vi "Sort Scan Parameters.vi"(8 "error in (no error)":errorcluster, 11 "SweepControl":refnum<class "SweepControl.lvclass">) -> (0 "error out":errorcluster, 1 "Sorted scan parameters":cluster{T1}[](array[cluster])=[{[{"Start"=0.14, "End"=-0.060000000000000005, "Step"=-0.060000000000000005, "Rate"=0.0, "wait (ms)"=10000, "Address"="Dev2/ao0", "channel"=1}]}, {[{"Start"=0.14, "End"=-0.060000000000000005, "Step"=-0.060000000000000005, "Rate"=0.0, "wait (ms)"=10000, "Address"="Dev2/ao0", "channel"=1}]}, {[{"Start"=0.14, "End"=-0.060000000000000005, "Step"=-0.060000000000000005, "Rate"=0.0, "wait (ms)"=10000, "Address"="Dev2/ao0", "channel"=1}, {"Start"=0.14, "End"=-0.060000000000000005, "Step"=-0.060000000000000005, "Rate"=0.0, "wait (ms)"=10000, "Address"="Dev2/ao0", "channel"=1}]}] {"?"."Rate" format="%.2f"; "?"."Step" format="%#_6p"; "?"."End" format="%#_6p"; "?"."Start" format="%#_6p"}, 2 "Sorted scan control":cluster{T3}[](array[cluster])=[{[{"Priority"=enum."Priority 0", "Scan name"=enum."DSA_Vsg2"}]}, {[{"Priority"=enum."Priority 1", "Scan name"=enum."DSA_Vamp"}]}, {[{"Priority"=enum."Priority 2", "Scan name"=enum."DSA_Vsg1"}, {"Priority"=enum."Priority 2", "Scan name"=enum."DSA_Vsg3"}]}], 3 "SweepControl":refnum<class "SweepControl.lvclass">)   [LabVIEW 2016, in "SweepControl.lvclass"]
uses:
  SweepControl.lvclass
  Typedefs/ScanControl.ctl
  Typedefs/Cluster - ScanControl.ctl
  Typedefs/Enum - Priority.ctl
  Typedefs/Enum - Action.ctl
  Typedefs/ScanParamters.ctl
  Typedefs/Cluster - ScanParamters.ctl
  SweepControl.lvclass/SweepControl.ctl
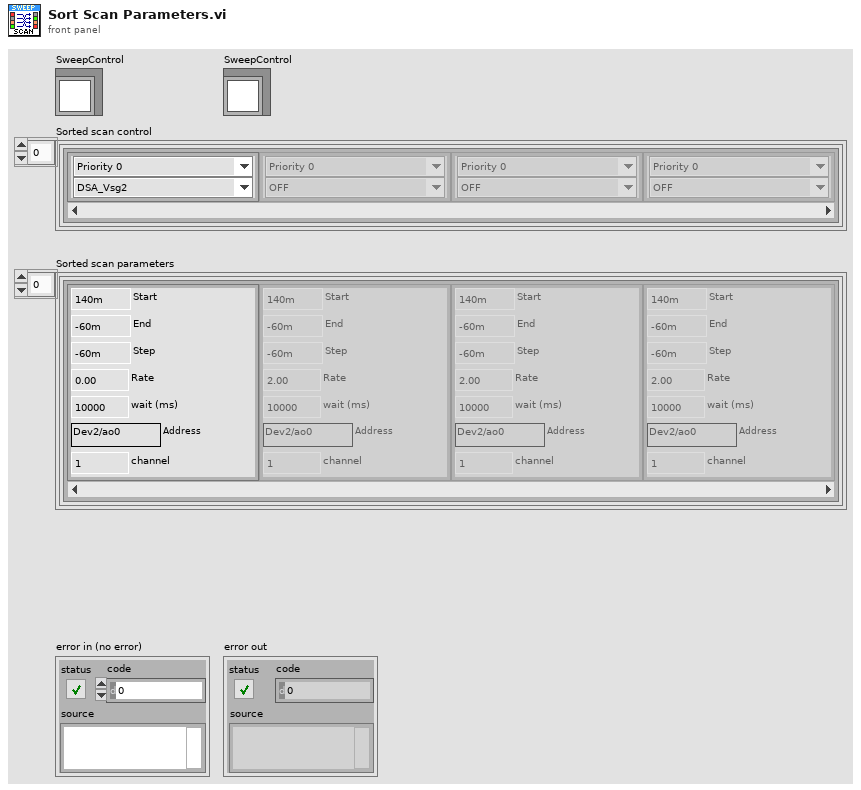
[diagram p1: front panel]
types:
  T1 = typedef "SweepControl.lvclass/ScanParamters.ctl" = T2[]
  T2 = typedef "SweepControl.lvclass/Cluster - ScanParamters.ctl" = cluster{"Start":dbl, "End":dbl, "Step":dbl, "Rate":dbl, "wait (ms)":u32, "Address":string, "channel":i32}
  T3 = typedef "SweepControl.lvclass/ScanControl.ctl" = T4[]
  T4 = typedef "SweepControl.lvclass/Cluster - ScanControl.ctl" = cluster{"Priority":T5, "Scan name":T6}
  T5 = typedef "SweepControl.lvclass/Enum - Priority.ctl" = enum16{"Priority 0", "Priority 1", "Priority 2", "Priority 3", "Priority 4", "Priority 5"}
  T6 = typedef "SweepControl.lvclass/Enum - Action.ctl" = enum16{"OFF", "DSA_Vamp", "DSA_freq", "DSA_Vsg1", "DSA_Vsg2", "DSA_Vsg3", "DAQ_Vbg", "B_Field", "Humidity", "Temp", "MW_freq1", "MW_freq2", "MW_amplitude1", "MW_amplitude2"}
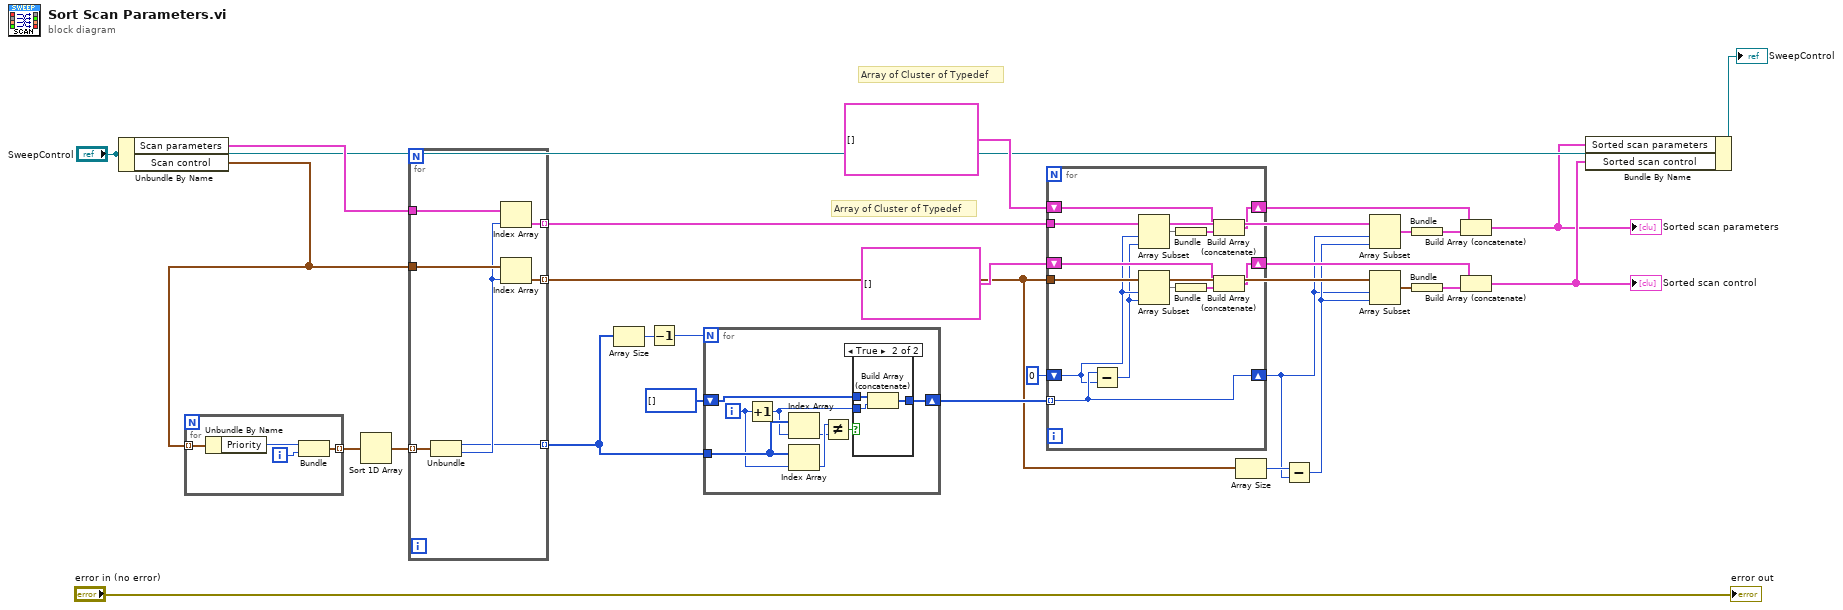
[diagram p0: block diagram]
diagram:
  # "Array of Cluster of Typedef"
  # "Array of Cluster of Typedef"
  n1 = Unbundle By Name("SweepControl") -> ("Scan parameters"=w7:T1, "Scan control"=w6:T3)
  n2 = for {
    tunnel: w6 -> [w29] mode=indexing
    tunnel: [w32] -> w28 mode=indexing
    i -> [w30]
    n3 = Unbundle By Name(w29) -> ("Priority"=w31:T5)
    n4 = Bundle("Priority"=w31, w30) -> (w32:cluster{"Priority":T5, i32})  [unwired: 1 in]
  }
  n5 = Sort 1D Array(array=w28) -> (sorted array=w27:cluster{"Priority":T5, i32}[])
  n6 = for {
    tunnel: w27 -> [w39] mode=indexing
    tunnel: w6 -> [w38]
    tunnel: [w37] -> w17 mode=indexing
    tunnel: w7 -> [w36]
    tunnel: [w35] -> w13 mode=indexing
    tunnel: [w33] -> w24 mode=indexing
    n7 = Unbundle(w39) -> ("Priority"=w33:T5, w34:i32)
    n8 = Index Array(array=w36, index=w34) -> (element=w35:T2)
    n9 = Index Array(array=w38, index=w34) -> (element=w37:T4)
  }
  n10 = Array Size(array=w24) -> (size(s)=w26:i32)
  n11 = Decrement(x=w26) -> (x-1=w25:i32)
  n12 = for {
    N: w25 -> [_]
    tunnel: w24 -> [w47]
    shift-right: [w43] -> w21
    shift-left: i32[] [] -> [w42]
    i -> [w40]
    n13 = Increment(x=w40) -> (x+1=w41:i32)
    n14 = Index Array(array=w47, index=w41) -> (element=w44:T5)
    n15 = Index Array(array=w47, index=w40) -> (element=w46:T5)
    n16 = Not Equal?(x=w46, y=w44) -> (x != y?=w45:bool)
    n17 = case shown="True" w45 {
      tunnel: [w48 w51] -> w43
      tunnel: w42 -> [w48 w50]
      tunnel: w41 -> [_ w49]
      frame False {
      }
      frame True {
        n18 = Build Array (concatenate)(w50, w49) -> (w51:i32[])
      }
    }
  }
  n19 = for {
    tunnel: w21 -> [w59] mode=indexing
    shift-right: [w64] -> w20
    shift-left: cluster{"Scan control":T3}[] [] -> [w63]
    tunnel: w17 -> [w62]
    shift-right: [w59] -> w11
    shift-left: 0 -> [w57]
    tunnel: w13 -> [w58]
    shift-right: [w54] -> w8
    shift-left: cluster{"Scan parameters":T1}[] [] -> [w53]
    n20 = Subtract(x=w59, y=w57) -> (x-y=w56:i32)
    n21 = Array Subset(array=w58, index=w57, length=w56) -> (w55:T2[])
    n22 = Array Subset(array=w62, index=w57, length=w56) -> (w61:T4[])
    n23 = Bundle(w55) -> (w52:cluster{T2[]})  [unwired: 1 in]
    n24 = Bundle(w61) -> (w60:cluster{T4[]})  [unwired: 1 in]
    n25 = Build Array (concatenate)(w53, w52) -> (w54:cluster{"Scan parameters":T1}[])
    n26 = Build Array (concatenate)(w63, w60) -> (w64:cluster{"Scan control":T3}[])
  }
  n27 = Array Size(array=w17) -> (size(s)=w18:i32)
  n28 = Subtract(x=w18, y=w11) -> (x-y=w12:i32)
  n29 = Array Subset(array=w13, index=w11, length=w12) -> (w14:T2[])
  n30 = Array Subset(array=w17, index=w11, length=w12) -> (w16:T4[])
  n31 = Bundle(w14) -> (w10:cluster{T2[]})  [unwired: 1 in]
  n32 = Bundle(w16) -> (w15:cluster{T4[]})  [unwired: 1 in]
  n33 = Build Array (concatenate)(w8, w10) -> (w2:cluster{"Scan parameters":T1}[])
  "Sorted scan parameters" <- w2
  n34 = Build Array (concatenate)(w20, w15) -> (w3:cluster{"Scan control":T3}[])
  "Sorted scan control" <- w3
  n35 = Bundle By Name(cluster="SweepControl", "Sorted scan parameters"=w2, "Sorted scan control"=w3) -> (→"SweepControl":refnum<class "SweepControl.lvclass">)
  "error out" <- "error in (no error)"
